vi "ReferencedVariables_ReadReferencedVariable_6x8x6_Singleton.vi"(5 "error in (no error)":errorcluster) -> (15 "ReplaceWithtypeDef":dbl, 19 "error out":errorcluster)   [LabVIEW 2016]
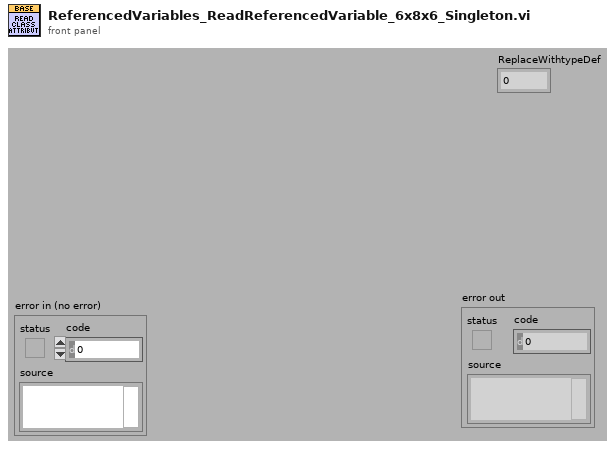
[diagram p1: front panel]
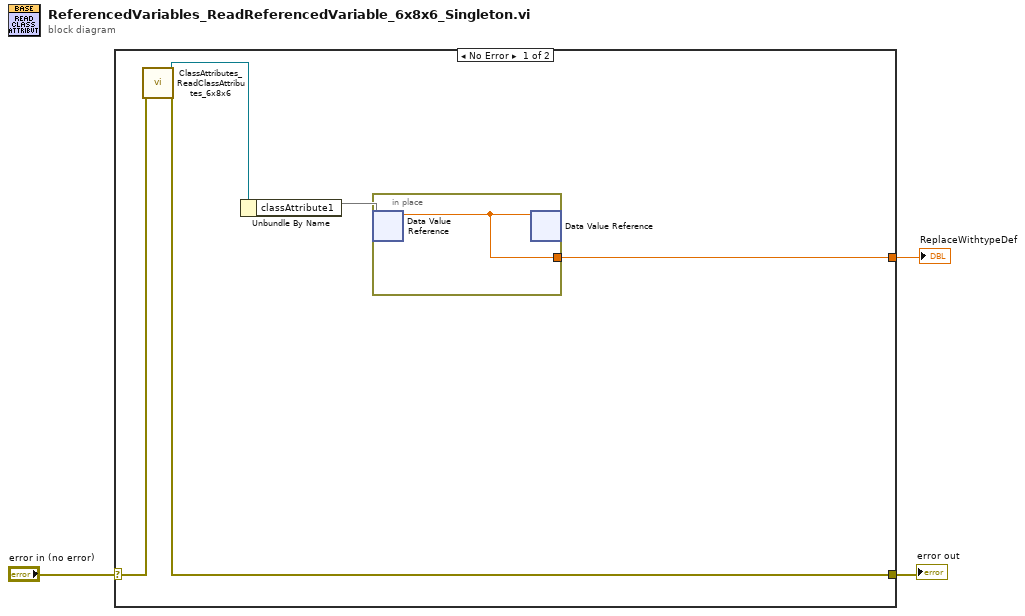
[diagram p0: block diagram]
diagram:
  n1 = case shown="No Error" "error in (no error)" {
    selector: "error in (no error)" -> [w8 w10]
    tunnel: [w6 w10] -> w2
    tunnel: [w4 _] -> w1
    frame No Error {
      n2 = call <resource>:"ClassAttributes_ReadClassAttributes_6x8x6.vi"("error in (no error)"=w8) -> ("reference out"=w5:refnum<class>, "error out"=w6:errorcluster)  [unwired: 17 in]
      n3 = Unbundle By Name(w5) -> ("classAttribute1"=w7)
      n4 = in-place {
        in-place-border: [w9] -> w4
        n5 = in-place-dvr #1(w7) -> (w9:dbl)  [unwired: 1 out]
        n6 = in-place-dvr #1(w9) -> ()  [unwired: 2 out]
      }
    }
    frame Error {
    }
  }
  "error out" <- w2
  "ReplaceWithtypeDef" <- w1
